vi "Register Configuration and Results.vi"(8 "error in":errorcluster, 10 "measurement plugin service in":refnum<class "Measurement Plugin Service.lvclass">, 11 "gRPC ID in":T1) -> (0 "error out":errorcluster, 2 "measurement plugin service out":refnum<class "Measurement Plugin Service.lvclass">, 3 "gRPC ID out":T1)   [LabVIEW 2020, in "Measurement Plugin Measurement Server.lvlib"]
uses:
  Measurement Plugin Measurement Server.lvlib
  <vilib>/gRPC/LabVIEW gRPC Library/grpc-lvsupport-release.lvlib
  Measurement Plugin Service/Measurement Plugin Service.lvclass
  <vilib>/gRPC/LabVIEW gRPC Library/Shared/grpcId.ctl
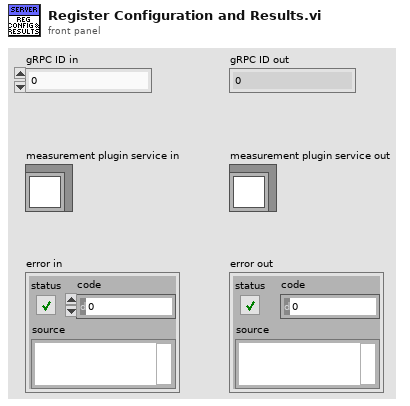
[diagram p1: front panel]
types:
  T1 = typedef "grpc-lvsupport-release.lvlib/grpcId.ctl" = u64
  T2 = typedef "Measurement Plugin Measurement Server.lvlib/Measurement Plugin Service.lvclass/Plugin Paths.ctl" = cluster{"get measurement details VI path":path, "get type specializations VI path":path, "get UI details VI path":path, "measurement logic VI path":path, "measurement configuration ctl path":path, "measurement results ctl path":path}
  T3 = typedef "grpc-lvsupport-release.lvlib/Enum Metadata.ctl" = cluster{"Version":i32, "Name":string, "Type Url":string, "Enum Values":string, "Allow Alias":bool}
  T4 = typedef "grpc-lvsupport-release.lvlib/Message Metadata.ctl" = cluster{"Version":i32, "Name":string, "Type Url":string, "Elements":T5[], "Has Oneof":bool}
  T5 = typedef "grpc-lvsupport-release.lvlib/Message Element Metadata.ctl" = cluster{"Field Name":string, "Embedded Message Name":string, "Protobuf Index":i32, "MessageElementType":T6, "Repeated":bool, "Is in Oneof":bool, "Oneof Container Name":string}
  T6 = typedef "grpc-lvsupport-release.lvlib/Message Element Type.ctl" = enum32{"Int32Value", "FloatValue", "DoubleValue", "BoolValue", "StringValue", "MessageValue", "Int64Value", "UInt32Value", "UInt64Value", "EnumValue", "Bytes", "Fixed64", "Fixed32", "SFixed64", "SFixed32", "SInt64", "SInt32"}
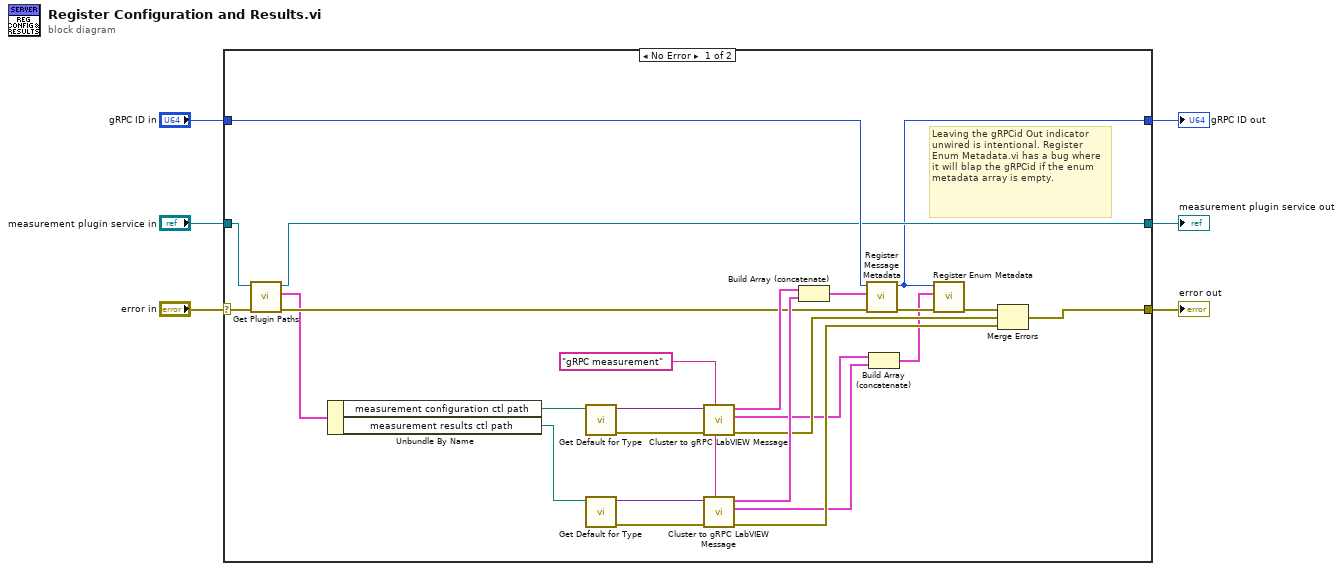
[diagram p0: block diagram]
diagram:
  n1 = case shown="No Error" "error in" {
    selector: "error in" -> [w18 w34]
    tunnel: [w10 w33] -> w3
    tunnel: [w28 w34] -> w6
    tunnel: "gRPC ID in" -> [w25 w33]
    tunnel: "measurement plugin service in" -> [w19 w32]
    tunnel: [w13 w32] -> w1
    frame No Error {
      w24 = "gRPC measurement" ("Package Name")
      # "Leaving the gRPCid Out indicator unwired is intentional. Register Enum Metadata.vi has a bug where it will blap the gRPCid if the enum metadata array is empty."
      n2 = call-dynamic "Get Plugin Paths.vi"("error in"=w18, "measurement plugin service in"=w19) -> ("error out"=w17:errorcluster, "plugin paths"=w16:T2, "measurement plugin service out"=w13:refnum<class "Measurement Plugin Service.lvclass">)  [unwired: 7 in]
      n3 = Unbundle By Name(w16) -> ("measurement configuration ctl path"=w15:path, "measurement results ctl path"=w14:path)
      n4 = call "Get Default for Type.vi"("path of type"=w15) -> ("error out"=w22:errorcluster, "default for type"=w23:variant)  [unwired: 9 in]
      n5 = call "Get Default for Type.vi"("path of type"=w14) -> ("error out"=w20:errorcluster, "default for type"=w21:variant)  [unwired: 9 in]
      n6 = call <vilib>:"Cluster to gRPC LabVIEW Message.vi"("Package Name"=w24, "error in"=w22, "Cluster"=w23) -> ("error out"=w26:errorcluster, "gRPC Enum Metadata out"=w9:T3[], "gRPC Message Metadata []"=w31:T4[])  [unwired: 6 in]
      n7 = call <vilib>:"Cluster to gRPC LabVIEW Message.vi"("Package Name"=w24, "error in"=w20, "Cluster"=w21) -> ("error out"=w27:errorcluster, "gRPC Enum Metadata out"=w8:T3[], "gRPC Message Metadata []"=w30:T4[])  [unwired: 6 in]
      n8 = Build Array (concatenate)(w31, w30) -> (w29:T4[])
      n9 = call <vilib>:"Register Message Metadata.vi"("error in"=w17, "Messages"=w29, "gRPCid in"=w25) -> ("error out"=w12:errorcluster, "gRPCid out"=w10:T1)  [unwired: 7 in]
      n10 = Build Array (concatenate)(w9, w8) -> (w7:T3[])
      n11 = call <vilib>:"Register Enum Metadata.vi"("error in"=w12, "Enum Metadata"=w7, "gRPCid in"=w10) -> ("error out"=w11:errorcluster)  [unwired: 7 in, 1 out]
      n12 = Merge Errors(w11, w26, w27) -> (w28:errorcluster)
    }
    frame Error {
    }
  }
  "error out" <- w6
  "gRPC ID out" <- w3
  "measurement plugin service out" <- w1
